vi "TrafficLight.vi"(4 "Serial Data":T1) -> (0 "Green":bool, 1 "Yellow":bool, 2 "Red":bool)   [LabVIEW 2025]
uses:
  Serial Data.ctl
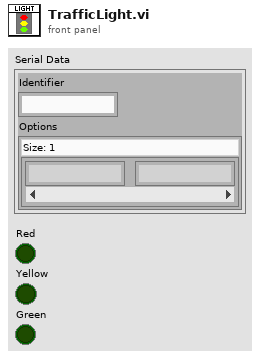
[diagram p1: front panel]
types:
  T1 = typedef "Serial Data.ctl" = cluster{"Identifier":string, "Options":map{string, string}}
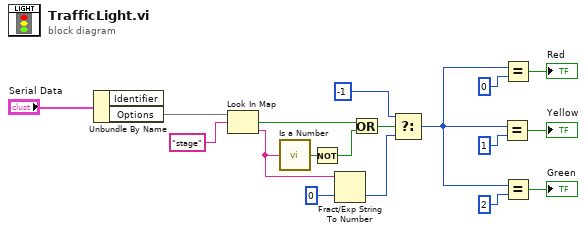
[diagram p0: block diagram]
diagram:
  n1 = Unbundle By Name("Serial Data") -> ("Options"=w18:map{string, string})  [unwired: 1 out]
  n2 = Look In Map(map=w18, key="stage") -> (key not found?=w16:bool, value=w13:string)  [unwired: 1 in]
  n3 = call "Is a Number.vi"("string"=w13) -> ("is a number?"=w15:bool)
  n4 = Not(x=w15) -> (.not. x?=w12:bool)
  n5 = Fract/Exp String To Number(string=w13, default (0 dbl)=0) -> (number=w14:i32)  [unwired: 2 in, 1 out]
  n6 = Or(x=w16, y=w12) -> (x .or. y?=w17:bool)
  n7 = Select(t=-1, s=w17, f=w14) -> (s? t:f=w4:i32)
  n8 = Equal?(x=w4, y=1) -> (x = y?=→"Yellow":bool)
  n9 = Equal?(x=w4, y=0) -> (x = y?=→"Red":bool)
  n10 = Equal?(x=w4, y=2) -> (x = y?=→"Green":bool)
